vi "SSH_spawn_model.vi"(9 "Joints":cluster{"Position (rad)":dbl, "Name":string}[](array[cluster]), 10 "Pose":T1, 11 "Settings":T2={"File Type"="sdf", "Model Source"="database", "Model Name"="", "Model Path"=""}) -> (3 "Command Sent":string)   [LabVIEW 2012]
panel:
  in  "Username":string="jed"
  in  "Host":string="130.64.87.197"
  out "standard output":string
  in  "password":string
  # "on the computer that is running the Gazebo simulator, run this command to start an empty world:\nroslaunch gazebo_ros empty_world.launch"
  # "\"Model Name\" is a label for your model\n\"Model Path\" is either the database item name (gas_station)\n       or the path to the model file (~/.gazebo/models/gas_station/model.sdf)\n\"File Type\" specifies the type of xml that the model file contains\n\"Model Source\" specifies where to find the model files"
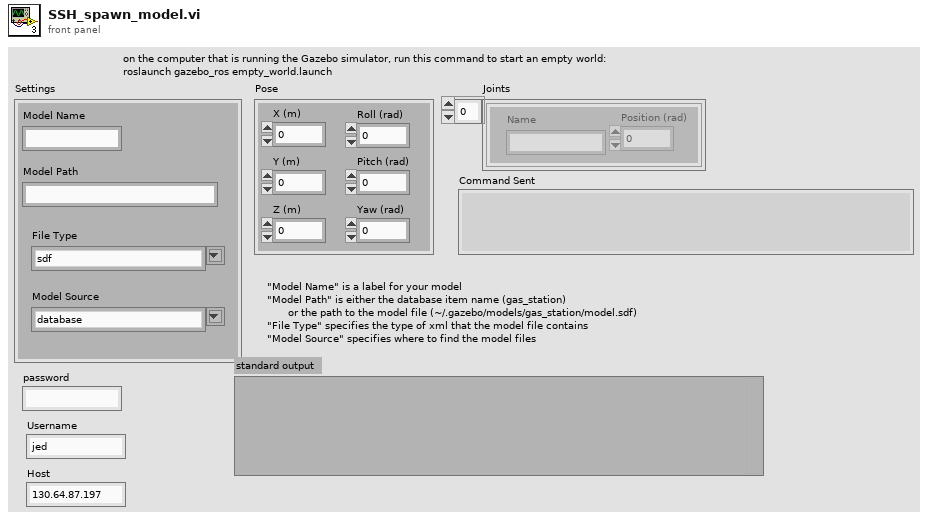
[diagram p1: front panel]
types:
  T1 = cluster{"X (m)":dbl, "Y (m)":dbl, "Z (m)":dbl, "Pitch (rad)":dbl, "Yaw (rad)":dbl, "Roll (rad)":dbl}
  T2 = cluster{"File Type":string, "Model Source":string, "Model Name":string, "Model Path":string}
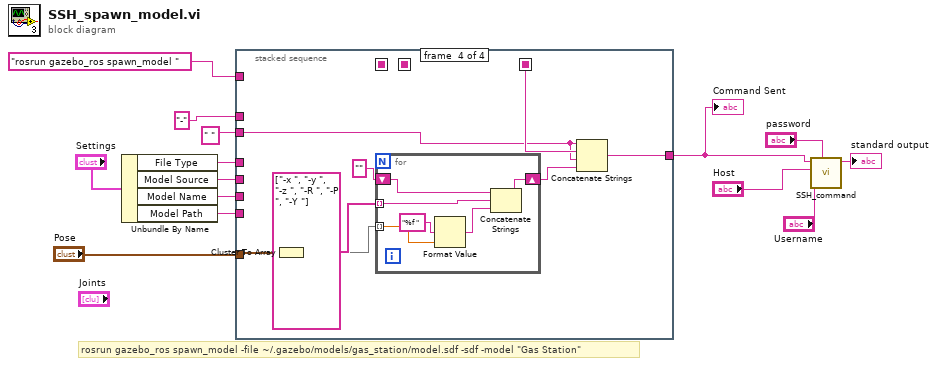
[diagram p0: block diagram]
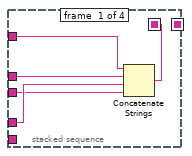
[diagram p2: hidden frame]
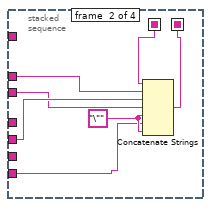
[diagram p3: hidden frame]
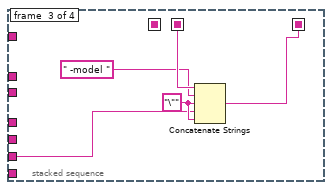
[diagram p4: hidden frame]
diagram:
  # "rosrun gazebo_ros spawn_model -file ~/.gazebo/models/gas_station/model.sdf -sdf -model \"Gas Station\""
  n1 = Unbundle By Name("Settings") -> ("File Type"=w13:string, "Model Source"=w9:string, "Model Name"=w7:string, "Model Path"=w8:string)
  n2 = stacked-sequence {
    seq-local: [w17 _ _ _] -> [_ w26 _ _]
    seq-local: [_ w22 _ _] -> [_ _ w31 _]
    seq-local: [_ _ w27 _] -> [_ _ _ w39]
    tunnel: w13 -> [w16 _ _ _]
    tunnel: "-" ("string") -> [w19 w25 _ _]
    tunnel: "rosrun gazebo_ros spawn_model " ("string") -> [w18 _ _ _]
    tunnel: " " ("string") -> [w15 w23 _ w34]
    tunnel: w9 -> [_ w24 _ _]
    tunnel: w8 -> [_ w20 _ _]
    tunnel: w7 -> [_ _ w28 _]
    tunnel: "Pose" -> [_ _ _ w38]
    tunnel: [_ _ _ w32] -> w5
    frame #0 {
      n3 = Concatenate Strings(w18, w19, w16, w15) -> (w17:string)
    }
    frame #1 {
      w21 = "\"" ("string")
      n4 = Concatenate Strings(w26, w25, w24, w23, w21, w20, w21) -> (w22:string)
    }
    frame #2 {
      w29 = "\"" ("string")
      n5 = Concatenate Strings(w31, " -model " ("string"), w29, w28, w29) -> (w27:string)
    }
    frame #3 {
      n6 = Cluster To Array(cluster=w38) -> (array=w36:dbl[])
      n7 = for {
        tunnel: string[] ["-x ", "-y ", "-z ", "-R ", "-P ", "-Y "] -> [w43] mode=indexing
        tunnel: w36 -> [w42] mode=indexing
        shift-right: [w45] -> w33
        shift-left: "" -> [w44]
        n8 = Format Value(format string="%f ", value (0)=w42) -> (output string=w41:string)  [unwired: 1 in]
        n9 = Concatenate Strings(w44, w43, w41) -> (w45:string)
      }
      n10 = Concatenate Strings(w34, w39, w34, w33) -> (w32:string)
    }
  }
  "Command Sent" <- w5
  n11 = call <userlib>:"SSH_command.vi"("password"="password", "Username"="Username", "Host"="Host", "Command(s) to Execute"=w5) -> ("standard output"=→"standard output":string)  [unwired: 5 in, 2 out]
